vi "write_ini_AdditionalSoftLimits.vi"(8 "error in (no error)":errorcluster caption="错误输入（无错误）", 10 "file ref in":T1, 11 "MotorSystem 输入":refnum<class "MotorSystem.lvclass">) -> (0 "error out":errorcluster caption="错误输出", 2 "file ref out":T1, 3 "MotorSystem 输出":refnum<class "MotorSystem.lvclass">)   [LabVIEW 2016, in "MotionControl.lvlib" / "MotorSystem.lvclass"]
uses:
  <userlib>/MotionControl/MotorSystem/MotorSystem.lvclass
  <vilib>/Utility/config.llb/Config Data RefNum.ctl
  <userlib>/MotionControl/MotorSystem/MotorSystem.lvclass/MotorSystem.ctl
  <vilib>/Utility/config.llb/Write Key (I32).vi
  <vilib>/Utility/config.llb/Write Key (String).vi
  <vilib>/Utility/config.llb/Write Key (Double).vi
  <vilib>/Utility/config.llb/NI_LVConfig.lvlib
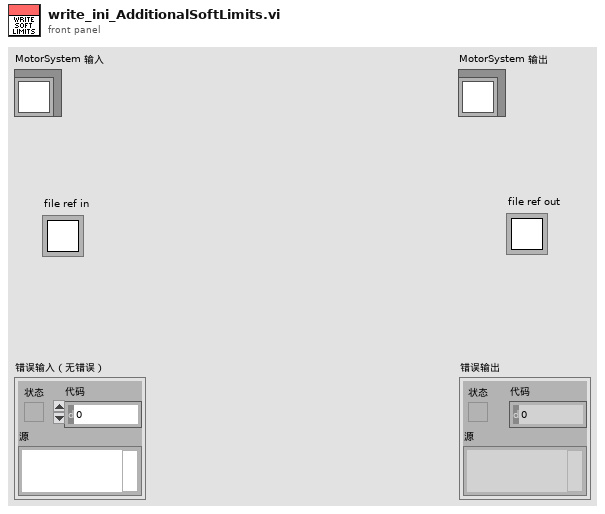
[diagram p1: front panel]
types:
  T1 = typedef "NI_LVConfig.lvlib/Config Data RefNum.ctl" = refnum<k1>
  T2 = cluster{"array for a soft limit":cluster{"dim name":string, "soft limit":cluster{"min":dbl, "max":dbl}}[]}[]
  T3 = cluster{"dim name":string, "soft limit":cluster{"min":dbl, "max":dbl}}[]
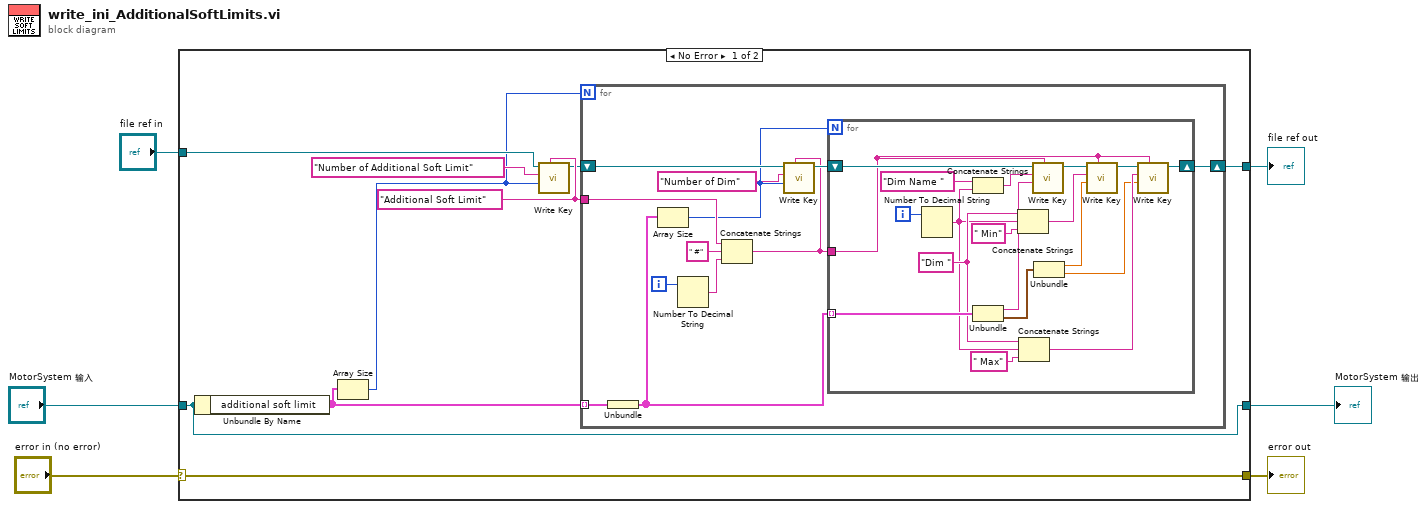
[diagram p0: block diagram]
diagram:
  n1 = case shown="No Error" "error in (no error)" {
    selector: "error in (no error)" -> [w15 w49]
    tunnel: [w15 w49] -> w5
    tunnel: [w14 w48] -> w3
    tunnel: "MotorSystem 输入" -> [w14 w48]
    tunnel: "file ref in" -> [w12 w47]
    tunnel: [w7 w47] -> w1
    frame No Error {
      w9 = "Additional Soft Limit"
      n2 = Unbundle By Name(w14) -> ("additional soft limit"=w13:T2)
      n3 = Array Size(array=w13) -> (size(s)=w10:i32)
      n4 = call-poly <vilib>:"Write Key.vi"("section"=w9, "value"=w10, "key"="Number of Additional Soft Limit", "refnum"=w12) -> ("refnum out"=w8:T1)  [unwired: 5 in, 2 out]
      n5 = for {
        N: w10 -> [_]
        tunnel: w13 -> [w27] mode=indexing
        tunnel: w9 -> [w25]
        shift-right: [w16] -> w7
        shift-left: w8 -> [w21]
        i -> [w22]
        n6 = Unbundle(w27) -> ("array for a soft limit"=w26:T3)
        n7 = Array Size(array=w26) -> (size(s)=w18:i32)
        n8 = Number To Decimal String(number=w22) -> (decimal integer string=w23:string)  [unwired: 1 in]
        n9 = Concatenate Strings(w25, " #", w23) -> (w17:string)
        n10 = call-poly <vilib>:"Write Key.vi"("section"=w17, "value"=w18, "key"="Number of Dim", "refnum"=w21) -> ("refnum out"=w20:T1)  [unwired: 5 in, 2 out]
        n11 = for {
          N: w18 -> [_]
          tunnel: w26 -> [w46] mode=indexing
          shift-right: [w28] -> w16
          shift-left: w20 -> [w44]
          tunnel: w17 -> [w29]
          i -> [w43]
          w34 = "Dim "
          n12 = Number To Decimal String(number=w43) -> (decimal integer string=w33:string)  [unwired: 1 in]
          n13 = Concatenate Strings("Dim Name ", w33) -> (w41:string)
          n14 = Unbundle(w46) -> ("dim name"=w40:string, "soft limit"=w45:cluster{"min":dbl, "max":dbl})
          n15 = Concatenate Strings(w34, w33, " Min") -> (w37:string)
          n16 = Concatenate Strings(w34, w33, " Max") -> (w31:string)
          n17 = call-poly <vilib>:"Write Key.vi"("section"=w29, "value"=w40, "key"=w41, "refnum"=w44) -> ("refnum out"=w39:T1)  [unwired: 5 in, 2 out]
          n18 = Unbundle(w45) -> ("min"=w36:dbl, "max"=w30:dbl)
          n19 = call-poly <vilib>:"Write Key.vi"("section"=w29, "value"=w36, "key"=w37, "refnum"=w39) -> ("refnum out"=w35:T1)  [unwired: 5 in, 2 out]
          n20 = call-poly <vilib>:"Write Key.vi"("section"=w29, "value"=w30, "key"=w31, "refnum"=w35) -> ("refnum out"=w28:T1)  [unwired: 5 in, 2 out]
        }
      }
    }
    frame Error {
    }
  }
  "error out" <- w5
  "MotorSystem 输出" <- w3
  "file ref out" <- w1
